vi "Create Dir if Non-Existant_with strip first.vi"(7 "Strip Path First [F]":bool, 8 "error in (no error)":errorcluster, 9 "permissions (0777)":i16=511 format="%.0o", 11 "Directory Path":path) -> (0 "error out":errorcluster, 2 "Created Directories":path[](array[path]), 3 "dup Directory Path":path)   [LabVIEW 2023]
doc: "Will create all directories above and including the directory defined by the \"Directory Path\" input, if they do not already exist.\n\nDRW version: optionally strip path. This allows a file (rather than a folder) path to be passed in. Output path will still be = input path."
uses:
  <userlib>/_OpenG.lib/file/file.llb/openg_file.lvlib
panel:
  # "Create Dir if Non-Existant.vi\n\nWill create all directories above and including the directory defined by the \"Directory Path\" input, if they do not already exist.\n\nPlease visit http://www.OpenG.org to learn about the\nOpen Source LabVIEW software movement.\n\nNOTICE -- YOU MUST LEAVE THIS NOTICE IN PLACE.  PER THE TERMS OF THE LICENSE BELOW, YOU MAY SUBLICENSE THIS SOFTWARE \nIN ANY WAY THAT DOES NOT CONFLICT WITH THIS LICENSE.\n\n### BSD License (http://www.opensource.org/licenses/bsd-license.php) Begin ###\n \nCopyright (c) 2002-2006, Jim Kring <jim@jimkring.com>\nCopyright (c) 2002, Cal-Bay Systems, Inc. <info@calbay.com>\n\nAll rights reserved.\n\nRedistribution and use in source and binary forms, with or without modification, are permitted provided that the following conditions are met:\n\n    * Redistributions of source code must retain the above copyright notice, this list of conditions and the following disclaimer.\n    * Redistributions in binary form must reproduce the above copyright notice, this list of conditions and the following disclaimer in the \n       documentation and/or other materials provided with the distribution.\n    * Neither the name of SciWare, James Kring, Inc., nor the names of its contributors may be used to endorse or promote products derived \n       from this software without specific prior written permission.\n\nTHIS SOFTWARE IS PROVIDED BY THE COPYRIGHT HOLDERS AND CONTRIBUTORS \"AS IS\" AND ANY EXPRESS OR IMPLIED WARRANTIES, \nINCLUDING, BUT NOT LIMITED TO, THE IMPLIED WARRANTIES OF MERCHANTABILITY AND FITNESS FOR A PARTICULAR PURPOSE ARE \nDISCLAIMED. IN NO EVENT SHALL THE COPYRIGHT OWNER OR CONTRIBUTORS BE LIABLE FOR ANY DIRECT, INDIRECT, INCIDENTAL,\n SPECIAL, EXEMPLARY, OR CONSEQUENTIAL DAMAGES (INCLUDING, BUT NOT LIMITED TO, PROCUREMENT OF SUBSTITUTE GOODS OR \nSERVICES; LOSS OF USE, DATA, OR PROFITS; OR BUSINESS INTERRUPTION) HOWEVER CAUSED AND ON ANY THEORY OF LIABILITY, \nWHETHER IN CONTRACT, STRICT LIABILITY, OR TORT (INCLUDING NEGLIGENCE OR OTHERWISE) ARISING IN ANY WAY OUT OF THE USE \nOF THIS SOFTWARE, EVEN IF ADVISED OF THE POSSIBILITY OF SUCH DAMAGE.\n\n### BSD License End ###"
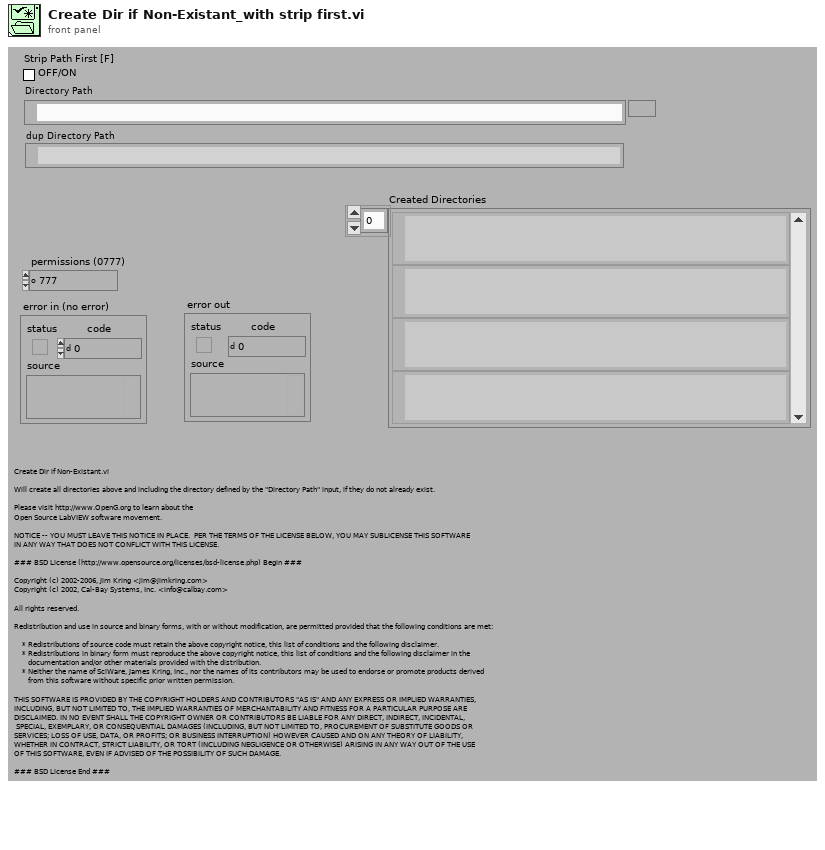
[diagram p1: front panel]
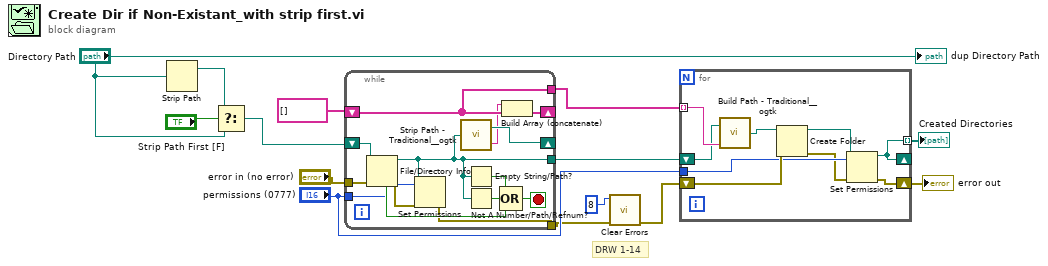
[diagram p0: block diagram]
diagram:
  # "DRW 1-14"
  n1 = Strip Path(path="Directory Path") -> (stripped path=w6:path)  [unwired: 1 out]
  n2 = Select(t=w6, s="Strip Path First [F]", f="Directory Path") -> (s? t:f=w8:path)
  n3 = while {
    shift-right: [w21] -> _
    shift-left: w8 -> [w28]
    shift-right: [w27] -> _
    shift-left: string[] [] -> [w26]
    tunnel: [w26] -> w12
    tunnel: [w19] -> w11
    tunnel: "permissions (0777)" -> [w18]
    tunnel: "error in (no error)" -> [w17]
    tunnel: [w15] -> w2
    stop <- w25 stop-if-true
    n4 = File/Directory Info(path=w28, error in=w17) -> (path out=w19:path, directory=w22:bool, error out=w16:errorcluster)  [unwired: 4 out]
    n5 = Set Permissions(7:w18, 8:w16, 11:w19) -> (0:w15:errorcluster)  [unwired: 2 in, 1 out]
    n6 = call <userlib>:"Strip Path - Traditional__ogtk.vi"("path"=w19) -> ("stripped path"=w21:path, "name"=w20:string)
    n7 = Empty String/Path?(string/path=w19) -> (empty?=w24:bool)
    n8 = Not A Number/Path/Refnum?(number/path/refnum=w19) -> (NaN/Path/Refnum?=w23:bool)
    n9 = Compound Arithmetic op=OR(w24, w23, w22) -> (w25:bool)
    n10 = Build Array (concatenate)(w20, w26) -> (w27:string[])
  }
  n11 = call <vilib>:"Clear Errors.vi"("error in (no error)"=w2, "specific error code to clear (0: all)"=8) -> ("error out"=w1:errorcluster)  [unwired: 4 in, 1 out]
  n12 = for {
    tunnel: w12 -> [w37] mode=indexing
    shift-right: [w31] -> _
    shift-left: w11 -> [w36]
    shift-right: [w35] -> w13
    shift-left: w1 -> [w34]
    tunnel: "permissions (0777)" -> [w32]
    tunnel: [w31] -> w9 mode=indexing
    n13 = call <userlib>:"Build Path - Traditional__ogtk.vi"("name or relative path"=w37, "base path"=w36) -> ("appended path"=w33:path)
    n14 = Create Folder(path (use dialog)=w33, error in=w34) -> (created path=w30:path, error out=w29:errorcluster)  [unwired: 1 in, 1 out]
    n15 = Set Permissions(7:w32, 8:w29, 11:w30) -> (0:w35:errorcluster, 3:w31:path)  [unwired: 2 in]
  }
  "error out" <- w13
  "Created Directories" <- w9
  "dup Directory Path" <- "Directory Path"
